vi "Gray to Color.vi"(7 "Mode":T2(ring), 8 "error in":errorcluster, 11 "Image In":T1) -> (0 "error out":errorcluster, 3 "Image Out":T1(plugin-control))   [LabVIEW 2015]
uses:
  <vilib>/vision/Image Controls.llb/IMAQ Image.ctl
  <vilib>/vision/NI_Vision_Development_Module.lvlib
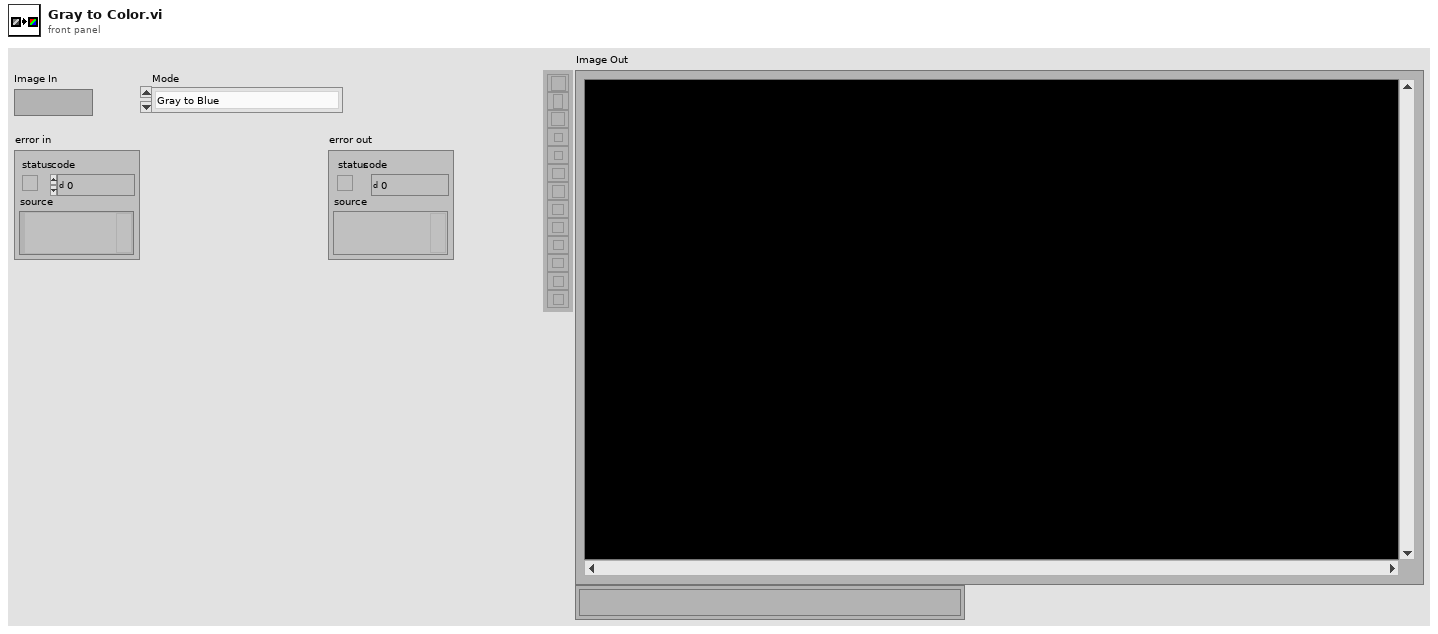
[diagram p1: front panel]
types:
  T1 = typedef "IMAQ Image.ctl" = refnum<image>
  T2 = enum16{"Gray to Blue", "Gray to Green", "Gray to Red", "Gray to Yellow", "Gray to Magenta", "Gray to Cyan"}
  T3 = typedef "Image Type" = u32
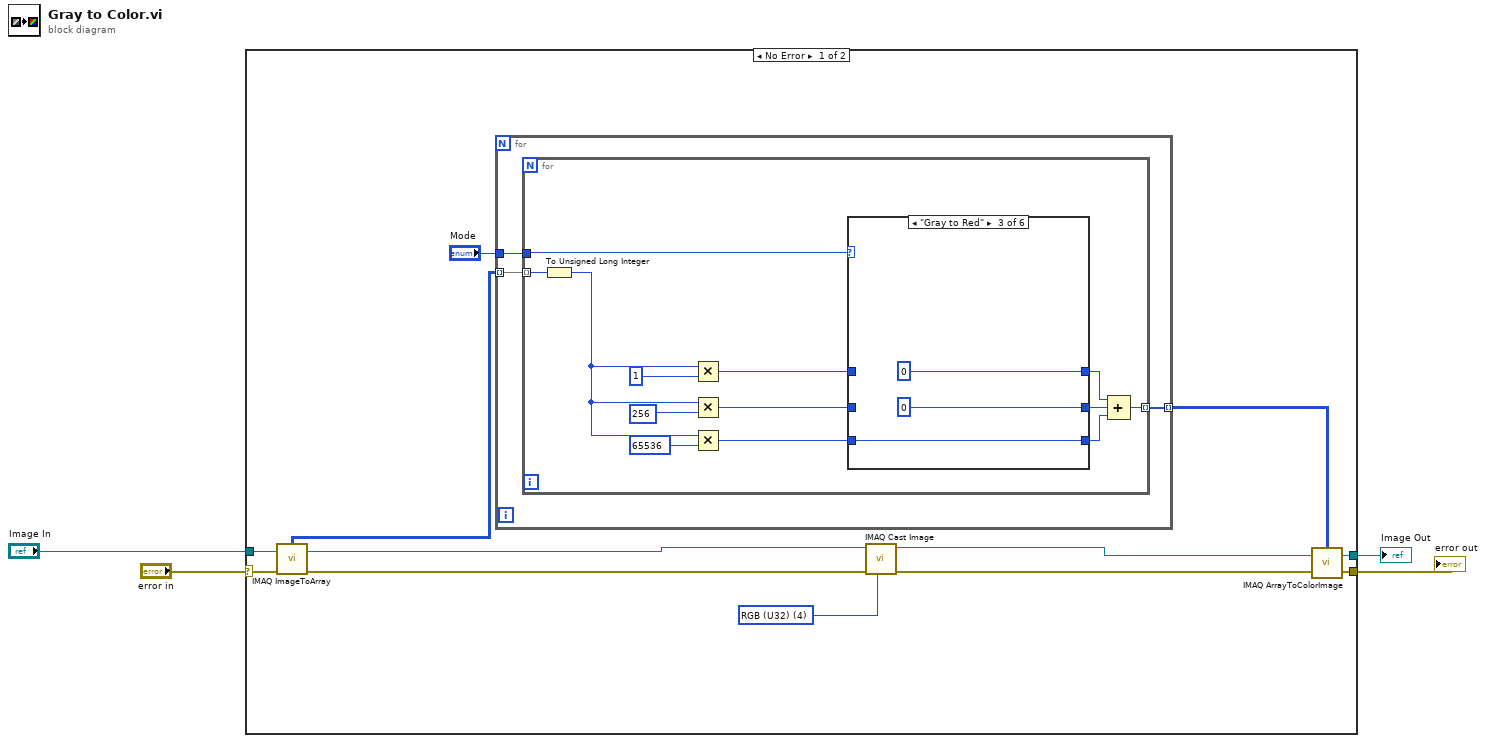
[diagram p0: block diagram]
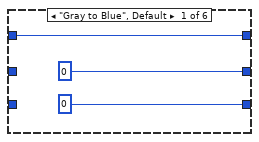
[diagram p2: hidden frame]
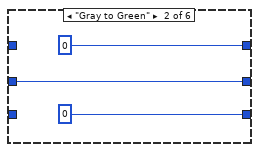
[diagram p3: hidden frame]
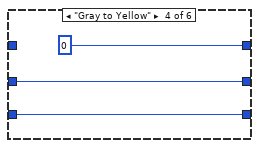
[diagram p4: hidden frame]
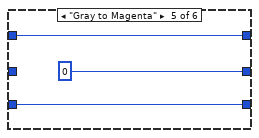
[diagram p5: hidden frame]
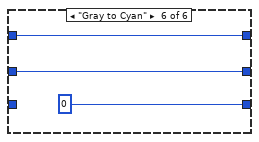
[diagram p6: hidden frame]
diagram:
  n1 = case shown="No Error" "error in" {
    selector: "error in" -> [w5 w50]
    tunnel: [w15 w51] -> w4
    tunnel: "Image In" -> [w10 w51]
    tunnel: [w6 w50] -> w3
    frame No Error {
      w11 = T3 4 items=["Grayscale (U8)", "Grayscale (I16)", "Grayscale (SGL)", "Complex (CSG)", "RGB (U32)", "HSL (U32)", "RGB (U64)", "Grayscale (U16)"] ("Image Type")
      n2 = call "IMAQ ImageToArray"("error in (no error)"=w5, "Image"=w10) -> ("error out"=w8:errorcluster, "Image Pixels (U8)"=w13:u8[][])  [unwired: 2 in, 3 out]
      n3 = for {
        tunnel: w13 -> [w18] mode=indexing
        tunnel: [w17] -> w14 mode=indexing
        tunnel: "Mode" -> [w16]
        n4 = for {
          tunnel: w18 -> [w31] mode=indexing
          tunnel: [w29] -> w17 mode=indexing
          tunnel: w16 -> [w28]
          n5 = To Unsigned Long Integer(number=w31) -> (unsigned 32bit integer=w30:u32)
          n6 = Multiply(x=w30, y=1) -> (x*y=w24:u32)
          n7 = Multiply(x=w30, y=256) -> (x*y=w23:u32)
          n8 = Multiply(x=w30, y=65536) -> (x*y=w22:u32)
          n9 = case shown="\"Gray to Red\"" w28 {
            tunnel: [w34 u32 0 u32 0 u32 0 w45 w49] -> w27
            tunnel: [u32 0 w37 u32 0 w43 u32 0 w48] -> w26
            tunnel: [u32 0 u32 0 w40 w42 w46 u32 0] -> w25
            tunnel: w24 -> [w34 _ _ _ w45 w49]
            tunnel: w23 -> [_ w37 _ w43 _ w48]
            tunnel: w22 -> [_ _ w40 w42 w46 _]
            frame "Gray to Blue", Default {
            }
            frame "Gray to Green" {
            }
            frame "Gray to Red" {
            }
            frame "Gray to Yellow" {
            }
            frame "Gray to Magenta" {
            }
            frame "Gray to Cyan" {
            }
          }
          n10 = Compound Arithmetic op=ADD(w27, w26, w25) -> (w29:u32)
        }
      }
      n11 = call "IMAQ Cast Image"("Image Type"=w11, "error in (no error)"=w8, "Image Src"=w10) -> ("error out"=w7:errorcluster, "Image Dst Out"=w9:T1)  [unwired: 7 in]
      n12 = call "IMAQ ArrayToColorImage"("Image Pixels (U32)"=w14, "Image"=w9, "error in (no error)"=w7) -> ("Image Out"=w15:T1, "error out"=w6:errorcluster)  [unwired: 2 in]
    }
    frame Error {
    }
  }
  "Image Out" <- w4
  "error out" <- w3
